vi "LED Visual Confirmation.vi"() -> (3 "Pass":bool)   [LabVIEW 2015]
panel:
  in  "Fail":bool
  in  "Pass":bool
  # "Confirm that all LEDs are on."
  # "Confirma que todos los LEDs \nestan encendidos"
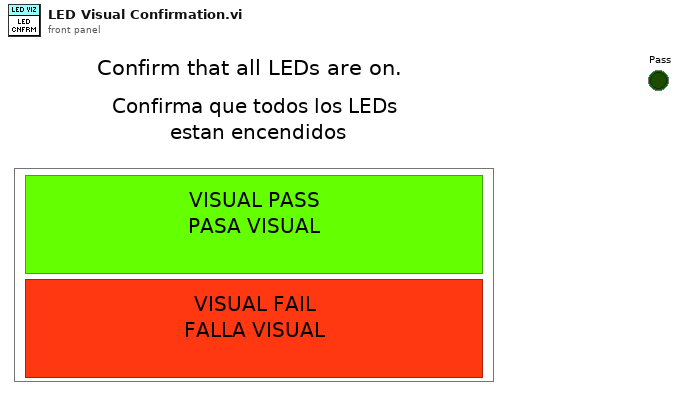
[diagram p1: front panel]
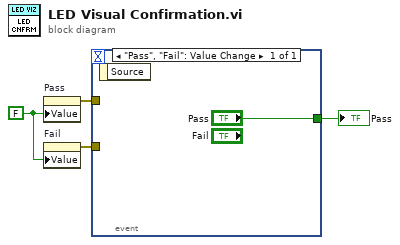
[diagram p0: block diagram]
diagram:
  w3 = FALSE ("Pass")
  n1 = property on="Pass" class="Bool (strict)"("Value"=w3) -> (error out=w2:errorcluster)  [unwired: 2 in, 1 out]
  n2 = property on="Fail" class="Bool (strict)"("Value"=w3) -> (error out=w1:errorcluster)  [unwired: 2 in, 1 out]
  n3 = event shown="[0] \"Pass\", \"Fail\": Value Change" {
    selector: _ -> [_]
    dyn-events: _ -> [_]
    timeout: _ -> [_]
    tunnel: ["Pass"] -> w4
    tunnel: w2 -> [_]
    tunnel: w1 -> [_]
    event "Pass", "Fail": Value Change {
      n4 = event-data() -> ()  [unwired: 1 in, 1 out]
    }
  }
  "Pass" <- w4
